vi "TCP Write Length and Data (2D Array DBL).vi"(8 "Error In":errorcluster, 9 "Timeout":i32=1000, 10 "Data":dbl[][](array[numeric]), 11 "connection ID":refnum<k5>) -> (0 "Error Out":errorcluster, 3 "connection ID out":refnum<k5>)   [LabVIEW 2022 SP3]
doc: "This software is licensed for use under the “MIT License\"\nCopyright (c) 2019 Scott Hannahs, sth@alum.mit.edu\n\nPermission is hereby granted, free of charge, to any person obtaining a copy of this software and associated documentation files (the \"Software\"), to deal in the Software without restriction, including without limitation the rights to use, copy, modify, merge, publish, distribute, sublicense, and/or sell copies of the Software, and to permit persons to whom the Software is furnished to do so, subject to the following conditions: The above copyright notice and this permission notice shall be included in all copies or substantial portions of the Software.\n\nTHE SOFTWARE IS PROVIDED \"AS IS\", WITHOUT WARRANTY OF ANY KIND, EXPRESS OR IMPLIED, INCLUDING BUT NOT LIMITED TO THE WARRANTIES OF MERCHANTABILITY, FITNESS FOR A PARTICULAR PURPOSE AND NONINFRINGEMENT. IN NO EVENT SHALL THE AUTHORS OR COPYRIGHT HOLDERS BE LIABLE FOR ANY CLAIM, DAMAGES OR OTHER LIABILITY, WHETHER IN AN ACTION OF CONTRACT, TORT OR OTHERWISE, ARISING FROM, OUT OF OR IN CONNECTION WITH THE SOFTWARE OR THE USE OR OTHER DEALINGS IN THE SOFTWARE."
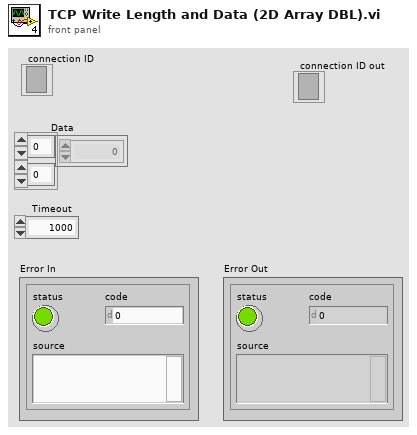
[diagram p1: front panel]
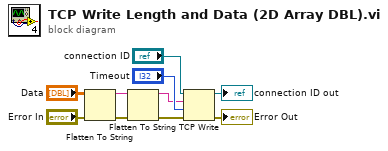
[diagram p0: block diagram]
diagram:
  n1 = Flatten To String(anything="Data", error in (no error)="Error In") -> (data string=w1:string, error out=w8:errorcluster)  [unwired: 2 in, 1 out]
  n2 = Flatten To String(anything=w1, error in (no error)=w8) -> (data string=w2:string, error out=w3:errorcluster)  [unwired: 2 in, 1 out]
  n3 = TCP Write(connection ID="connection ID", data in=w2, error in (no error)=w3, 9:"Timeout") -> (connection ID out=→"connection ID out":refnum<k5>, error out=→"Error Out":errorcluster)  [unwired: 1 out]
